vi "Array to Set.vi"(8 "error in":errorcluster, 11 "Array":variant) -> (0 "error out":errorcluster, 3 "Set":variant)   [LabVIEW 2020, in "openg_variant.lvlib"]
uses:
  openg_variant.lvlib
  Type Descriptor Enumeration.ctl
panel:
  # "EXPERIMENTAL"
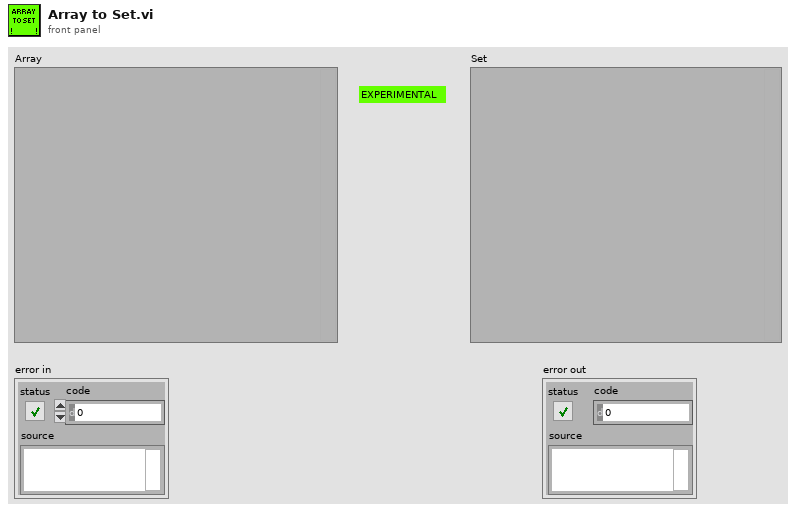
[diagram p1: front panel]
types:
  T1 = typedef "openg_variant.lvlib/Type Descriptor Enumeration.ctl" = enum8{"<Null>", "I8", "I16", "I32", "I64", "U8", "U16", "U32", "U64", "SGL", "DBL", "EXT", "CSG", "CDB", "CXT", "0x0F", "0x10", "0x11", "0x12", "0x13", "0x14", "Enum U8", "Enum U16", "Enum U32", "Enum U64", "SGL PQ", "DBL PQ", "EXT PQ", "CSG PQ", "CDB PQ", "CXT PQ", "0x1F", "0x20", "Boolean", "0x22", "0x23", "0x24", "0x25", "0x26", "0x27", "0x28", "0x29", "0x2A", "0x2B", "0x2C", "0x2D", "0x2E", "0x2F", "String", "0x31", "Path", "Pict", "0x34", "0x35", "0x36", "DAQ", "0x38", "0x39", "0x3A", "0x3B", "0x3C", "0x3D", "0x3E", "0x3F", "Array", "0x41", "0x42", "0x43", "0x44", "0x45", "0x46", "0x47", "0x48", "0x49", "0x4A", "0x4B", "0x4C", "0x4D", "0x4E", "0x4F", "Cluster", "0x51", "0x52", "Variant", "Waveform", "0x55", "0x56", "0x57", "0x58", "0x59", "0x5A", "0x5B", "0x5C", "0x5D", "0x5E", "Fixed Point", "0x60", "0x61", "0x62", "0x63", "0x64", "0x65", "0x66", "0x67", "0x68", "0x69", "0x6A", "0x6B", "0x6C", "0x6D", "0x6E", "0x6F", "Refnum", "0x71", "0x72", "Set Collection", "Map Collection"}
  T2 = typedef "openg_variant.lvlib/Type Descriptor.ctl" = i16[]
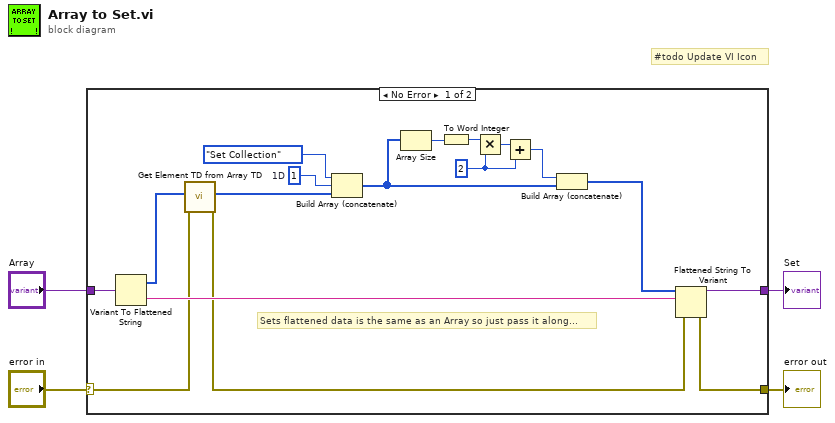
[diagram p0: block diagram]
diagram:
  # "#todo Update VI Icon"
  n1 = case shown="No Error" "error in" {
    selector: "error in" -> [w7 w22]
    tunnel: "Array" -> [w12 _]
    tunnel: [w11 _] -> w3
    tunnel: [w10 w22] -> w2
    frame No Error {
      w20 = i16 2 ("x")
      w14 = i16 1  # 1D
      # "Sets flattened data is the same as an Array so just pass it along..."
      n2 = Variant To Flattened String(Variant=w12) -> (data string=w13:string, 1:w9:i16[])
      n3 = call "Get Element TD from Array TD.vi"("error in (no error)"=w7, "Array Type Descriptor"=w9) -> ("error out"=w6:errorcluster, "Element Type Descriptor"=w8:T2)  [unwired: 8 in]
      n4 = Build Array (concatenate)(Type_Descriptor_Enumeration."Set Collection" ("Type Descriptor Enumeration"), w14, w8) -> (w16:T2)
      n5 = Array Size(array=w16) -> (size(s)=w15:i32)
      n6 = To Word Integer(number=w15) -> (16bit integer=w17:i16)
      n7 = Multiply(x=w17, y=w20) -> (x*y=w18:i16)
      n8 = Add(x=w18, y=w20) -> (x+y=w19:i16)
      n9 = Build Array (concatenate)(w19, w16) -> (w21:T2)
      n10 = Flattened String To Variant(4:w6, 6:w13, 7:w21) -> (0:w10:errorcluster, 3:w11:variant)
    }
    frame Error {
    }
  }
  "Set" <- w3
  "error out" <- w2
